vi "WFS Calc Reconstr Deviations.vi"(7 "Do Spherical Reference (No)":i32(ring) items=["Yes"=1, "No"=0], 8 "error in (no error)":errorcluster {"code" format="%.0x"}, 9 "Array Zernike Reconstruct":i32[](array[numeric]), 10 "Zernike Orders":i32 format="%.0g", 11 "instrument handle":refnum<visa-resource-name>) -> (0 "error out":errorcluster {"code" format="%.0x"}, 1 "Fit Err Stdev":dbl, 2 "Fit Err Mean":dbl, 3 "instrument handle out":refnum<visa-resource-name>)   [LabVIEW 2020]
doc: "This VI calculates the reconstructed spot deviations based on the calculated Zernike coefficients.\n\nNote: This VI needs to run prior to WFS Calc Wavefront.vi when the reconstructed or difference Wavefront should be calculated."
uses:
  WFS_32.dll
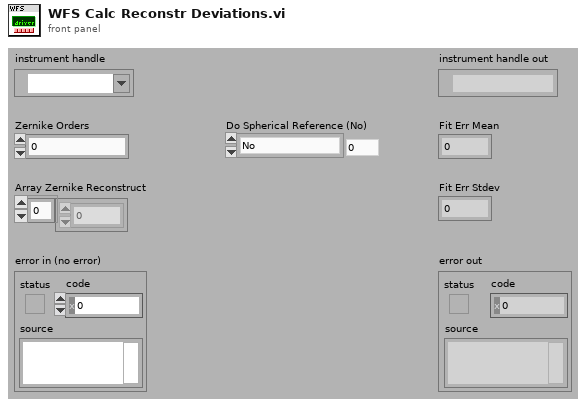
[diagram p1: front panel]
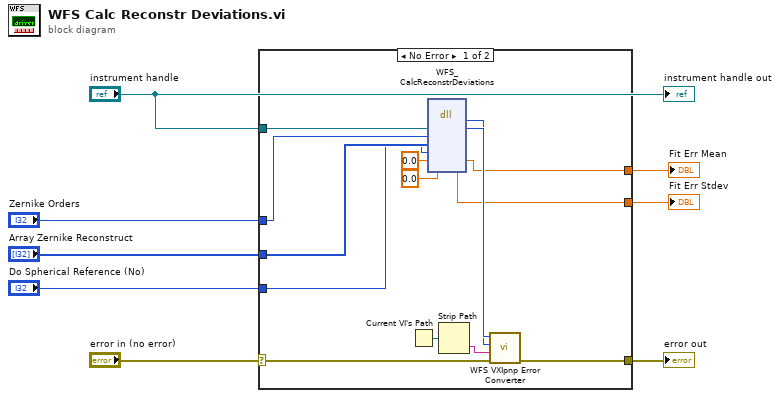
[diagram p0: block diagram]
diagram:
  n1 = case shown="No Error" "error in (no error)" {
    selector: "error in (no error)" -> [w17 w23]
    tunnel: [w16 w23] -> w8
    tunnel: "instrument handle" -> [w21 _]
    tunnel: "Zernike Orders" -> [w15 _]
    tunnel: "Array Zernike Reconstruct" -> [w14 _]
    tunnel: "Do Spherical Reference (No)" -> [w13 _]
    tunnel: [w11 _] -> w2
    tunnel: [w9 _] -> w1
    frame No Error {
      n2 = Current VI's Path() -> (path=w22:path)
      n3 = dll-call lib="WFS_*.*" fn="WFS_CalcReconstrDeviations"("Instrument Handle"=w21, "Zernike Orders"=w15, "Array Zernike Reconstruct"=w14, "Do Spherical Reference"=w13, "Fit Err Mean"=0.0, "Fit Err Stdev"=0.0) -> (w19:i32, "Instrument Handle"=w20:u32, "Fit Err Mean"=w11:dbl, "Fit Err Stdev"=w9:dbl)  [unwired: 6 in, 2 out]
      n4 = Strip Path(path=w22) -> (name=w18:string)  [unwired: 1 out]
      n5 = call "WFS VXIpnp Error Converter.vi"("error in (no error)"=w17, "Name Of VI (\"\")"=w18, "CVI Error Code (0)"=w19, "instrument handle"=w20) -> ("error out"=w16:errorcluster)  [unwired: 6 in, 1 out]
    }
    frame Error {
    }
  }
  "error out" <- w8
  "Fit Err Mean" <- w2
  "Fit Err Stdev" <- w1
  "instrument handle out" <- "instrument handle"
